vi "Part.b.vi"() -> ()   [LabVIEW 2013]
uses:
  <userlib>/labvvis/New Image/New Image (Grey).vi
  <userlib>/labvvis/labvvis.lvlib
panel:
  out "scissor":bool
  out "rock":bool
  out "paper":bool
  out "scissor_column_counter":u8
  out "paper_colum_counter":u8
  out "rock":u8
  out "Error":string
  in  "stop":bool
  in  "Threshold":u8(slide)=128 scale=0.0..255.0
  out "Output":picture
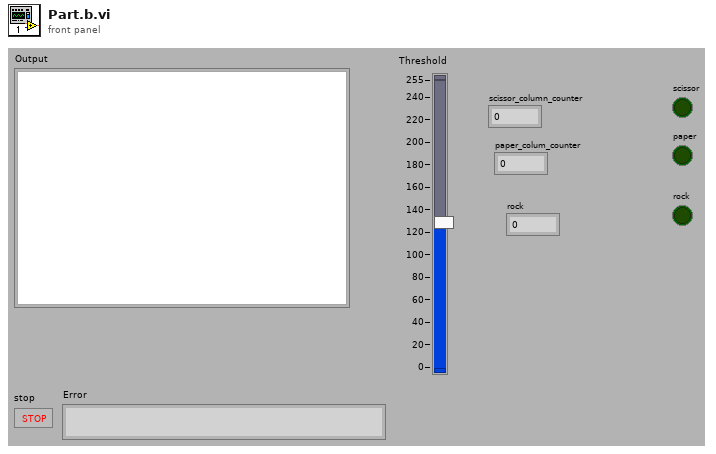
[diagram p1: front panel]
types:
  T1 = typedef "labvvis.lvlib/VVIS Image.ctl" = cluster{"Image ID":i16, "Channel ID":i16}
  T2 = typedef "imagedata.ctl" = cluster{"image type":i32, "image depth":i32, "image":u8[], "mask":u8[], "colors":u32[], "Rectangle":cluster{"left":i16, "top":i16, "right":i16, "bottom":i16}}
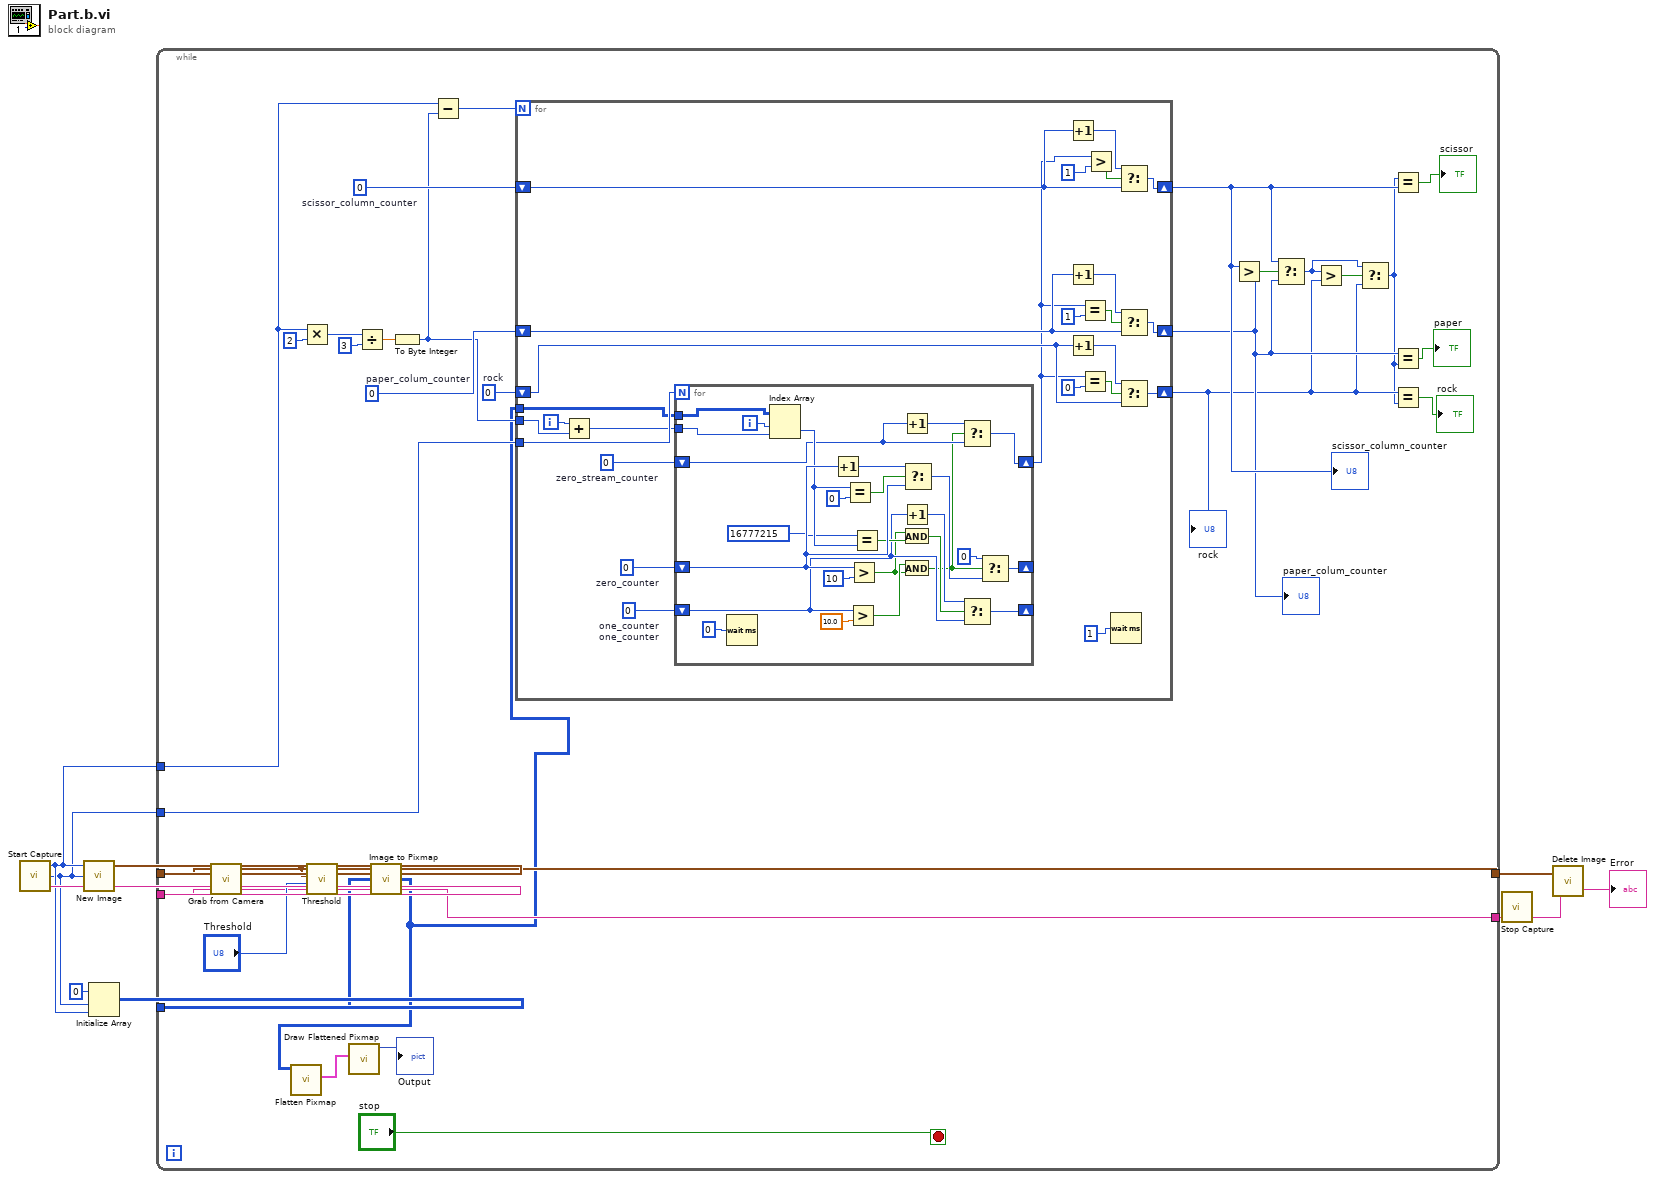
[diagram p0: block diagram]
diagram:
  n1 = call <userlib>:"Start Capture.vi"() -> ("Error"=w8:string, "Height"=w1:i32, "Width"=w2:i32)  [unwired: 3 in]
  n2 = call-poly <userlib>:"New Image.vi"("Error"=w8, "Height"=w1, "Width"=w2) -> ("Error"=w7:string, "VVIS Image"=w9:T1)  [unwired: 1 in]
  n3 = Initialize Array(0, w1, w2) -> (w10:i32[][])
  n4 = while {
    tunnel: w10 -> [w36]
    tunnel: w9 -> [w43]
    tunnel: w7 -> [w42]
    tunnel: [w37] -> w6
    tunnel: [w35] -> w5
    tunnel: w2 -> [w18]
    tunnel: w1 -> [w17]
    stop <- "stop" stop-if-true
    w28 = u8 0  # rock
    w29 = u8 0  # paper_colum_counter
    w30 = u8 0  # scissor_column_counter
    n5 = call <userlib>:"Grab from Camera.vi"("Error"=w42, "Image"=w43) -> ("Error"=w39:string, "Image"=w41:T1)  [unwired: 1 in, 1 out]
    n6 = Multiply(x=w18, y=i16 2) -> (x*y=w33:i32)
    n7 = call <userlib>:"Threshold.vi"("Error"=w39, "Threshold"="Threshold", "Output Image"=w41, "Input Image"=w41) -> ("Error"=w38:string, "Input Image"=w40:T1)  [unwired: 1 out]
    n8 = Divide(x=w33, y=i16 3) -> (x/y=w27:dbl)
    n9 = call <userlib>:"Image to Pixmap.vi"("Error"=w38, "Output Pixmap"=w36, "Image"=w40) -> ("Error"=w35:string, "Output Pixmap"=w12:u32[][], "Image"=w37:T1)
    n10 = call <vilib>:"Flatten Pixmap.vi"("24-bit pixmap"=w12) -> ("image data"=w13:T2)  [unwired: 10 in]
    n11 = call <vilib>:"Draw Flattened Pixmap.vi"("image data"=w13) -> ("new picture"=→"Output":picture)  [unwired: 8 in]
    n12 = To Byte Integer(number=w27) -> (8bit integer=w26:i8)
    n13 = Subtract(x=w18, y=w26) -> (x-y=w31:i32)
    n14 = for {
      N: w31 -> [_]
      tunnel: w17 -> [w71]
      tunnel: w12 -> [w70]
      tunnel: w26 -> [w68]
      shift-right: [w59] -> w22
      shift-left: w30 -> [w61]
      shift-right: [w55] -> w21
      shift-left: w29 -> [w57]
      shift-right: [w51] -> w20
      shift-left: w28 -> [w53]
      i -> [w69]
      w64 = 0  # zero_stream_counter
      w65 = u8 0  # one_counter one_counter
      w66 = u8 0  # zero_counter
      n15 = Add(x=w69, y=w68) -> (x+y=w67:i32)
      n16 = for {
        N: w71 -> [_]
        tunnel: w70 -> [w90]
        tunnel: w67 -> [w73]
        shift-right: [w77] -> _
        shift-left: w66 -> [w94]
        shift-right: [w87] -> _
        shift-left: w65 -> [w85]
        shift-right: [w82] -> w49
        shift-left: w64 -> [w83]
        i -> [w97]
        n17 = Wait (ms)(milliseconds to wait=u32 0) -> ()  [unwired: 1 out]
        n18 = Index Array(array=w90, index (row)=w97, index (col)=w73) -> (element=w92:u32)
        n19 = Increment(x=w94) -> (x+1=w95:u8)
        n20 = Equal?(x=w92, y=u8 0) -> (x = y?=w75:bool)
        n21 = Greater?(x=w85, y=10.0) -> (0:w81:bool)
        n22 = Greater?(x=w94, y=u8 10) -> (0:w80:bool)
        n23 = Equal?(x=u32 16777215, y=w92) -> (x = y?=w91:bool)
        n24 = Increment(x=w83) -> (x+1=w84:i32)
        n25 = Increment(x=w85) -> (x+1=w88:u8)
        n26 = And(x=w80, y=w91) -> (x .and. y?=w89:bool)
        n27 = And(x=w81, y=w80) -> (x .and. y?=w74:bool)
        n28 = Select(t=w95, s=w75, f=w94) -> (s? t:f=w79:u8)
        n29 = Select(t=w84, s=w74, f=w83) -> (s? t:f=w82:i32)
        n30 = Select(t=w88, s=w89, f=w85) -> (s? t:f=w87:u8)
        n31 = Select(t=u8 0, s=w74, f=w79) -> (s? t:f=w77:u8)
      }
      n32 = Increment(x=w61) -> (x+1=w60:u8)
      n33 = Increment(x=w57) -> (x+1=w56:u8)
      n34 = Increment(x=w53) -> (x+1=w52:u8)
      n35 = Equal?(x=w49, y=1) -> (x = y?=w58:bool)
      n36 = Equal?(x=w49, y=0) -> (x = y?=w54:bool)
      n37 = Greater?(x=w49, y=1) -> (0:w47:bool)
      n38 = Wait (ms)(milliseconds to wait=u32 1) -> ()  [unwired: 1 out]
      n39 = Select(t=w60, s=w47, f=w61) -> (s? t:f=w59:u8)
      n40 = Select(t=w56, s=w58, f=w57) -> (s? t:f=w55:u8)
      n41 = Select(t=w52, s=w54, f=w53) -> (s? t:f=w51:u8)
    }
    "rock" <- w20
    "paper_colum_counter" <- w21
    "scissor_column_counter" <- w22
    n42 = Greater?(x=w22, y=w21) -> (0:w25:bool)
    n43 = Select(t=w22, s=w25, f=w21) -> (s? t:f=w24:u8)
    n44 = Greater?(x=w24, y=w20) -> (0:w23:bool)
    n45 = Select(t=w24, s=w23, f=w20) -> (s? t:f=w19:u8)
    n46 = Equal?(x=w19, y=w22) -> (x = y?=→"scissor":bool)
    n47 = Equal?(x=w21, y=w19) -> (x = y?=→"paper":bool)
    n48 = Equal?(x=w20, y=w19) -> (x = y?=→"rock":bool)
  }
  n49 = call <userlib>:"Stop Capture.vi"("Error"=w5) -> ("Error"=w4:string)  [unwired: 4 in]
  n50 = call <userlib>:"Delete Image.vi"("Error"=w4, "Image"=w6) -> ("Error"=→"Error":string)  [unwired: 1 in]
